vi "Get Status.vi"(8 "error in (no error)":errorcluster, 10 "Header Contents in":T1={"FILENAME"=["FILENAME", "example.fits", "File name at acquisition"], "OBSERVER"=["OBSERVER", "ECHARPE", "PI name"], "PROGRID"=["PROGRID", "UNDEFINED", "Program ID"], "OBJECT"=["OBJECT", "UNDEFINED", "Object name"], "NIGHTDIR"=["NIGHTDIR", "C:\\Users\\Sparc4_2\\Desktop\\Software Echarpe\\Imagens", "Night directory name "], "CHANNEL"=["CHANNEL", "RED", "Instrument channel"], "INSTRUME"=["INSTRUME", "ECHARPE", "Instrument"], "NEXPSEQ"=["NEXPSEQ", "1", "Total number of exposures in sequence"], "SEQINDEX"=["SEQINDEX", "1", "Exposure index in the sequence"], "OBSTYPE"=["OBSTYPE", "BIAS", "Image type: OBJECT, BIAS, FLAT, ARC, DARK"], "READMOD"=["READMOD", "Normal", "Read out mode: fast, normal, slow"], "SHUTTER"=["SHUTTER", "CLOSED", "Shutter Mode (OPEN, CLOSED, or AUTO) "], "OPENSHT"=["OPENSHT", "50", "Time to open the shutter (ms) "], "CLOSESHT"=["CLOSESHT", "50", "Time to close the shutter (ms)"], "GAIN"=["GAIN", "3.38", "Gain (e-/ADU)"], "GAINERR "=["GAINERR", "0.05", " Gain error (e-/ADU)"], "RDNOISE"=["RDNOISE", "6.55", "Read noise (e-)"], "RNOISERR"=["RNOISERR", "0.02", "Read noise error (e-)"], "SKYFIBER"=["SKYFIBER", "OFF", "Sky fiber: ON or OFF"], "CALFIBER"=["CALFIBER", "OFF", "Calibration Fiber: ON or OFF"], "UTDATE"=["UTDATE", "2017-10-01T20", "UT date at start of exposure"], "LOCTIME"=["LOCTIME", "2017-10-01T17", "LT date at start of exposure"], "MJD"=["MJD", "58027.500000", "Modified Julian Date at start of exposure"], "OBSLON"=["OBSLON", "-45.57972", "Observatory East Longitude"], "OBSLAT"=["OBSLAT", "-22.53444", "Observatory Latitude"], "OBSALT"=["OBSALT", "1864.0", "Observatory elevation above sea level (m)"], "EXPTIME"=["EXPTIME", "1", "Exposure time (s)"], "TELRA"=["TELRA", "00:00:00.000", "TCS right ascension: HH:MM:SS.SSS"], "TELDEC"=["TELDEC", "+00:00:00.000", "TCS declination: +-DD:MM:SS.SSS"], "RA"=["RA", "00:00:00.000", "Requested right Ascension: HH:MM:SS.SSS"], "DEC"=["DEC", "+00:00:00.000", "Requested Declination: +- DD:MM:SS.SSS"], "RA_DEG"=["RA_DEG", "128.84946", "Requested Right Ascension (deg)"], "DEC_DEG"=["DEC_DEG", "+19.648717", "Requested Declination (deg)"], "EPOCH"=["EPOCH", "2000.00", "Epoch for Target coordinates"], "HA"=["HA", "+01:13:05.98", "Hour Angle (Sexagesimal)"], "HAD"=["HAD", "1.2183292", "Hour Angle (deg)"], "AIRMASS"=["AIRMASS", "1.085", "Mean airmass for the observation"], "AMSTART"=["AMSTART", "1.060", "Airmass at start of exposure"], "AMEND"=["AMEND", "1.114", "Airmass at end of exposure"], "XOFFSET"=["XOFFSET", "0.000000", "Telescope RA offset in arcsec"], "YOFFSET"=["YOFFSET", "0.000000", "Telescope DEC offset in arcsec"], "PA"=["PA", "14.6415392418", "Current Rotator Position Angle (degree)"], "CAMFOC"=["CAMFOC", "-3.53", "Camera focus position (mm)"], "TELFOC"=["TELFOC", "-3.53", "Telescope focus position (mm)"], "TCSUT"=["TCSUT", "23:17:24.8", "TCS Universal Time"], "MOONDIST"=["MOONDIST", "60.0", "Moon angular distance to object (deg)"], "MOONALT"=["MOONALT", "15.0", "Moon elevation above horizon (deg)"], "MONNPHAS"=["MOONPHAS", "30.0", "Moon phase (deg)"], "ADC"=["ADC", "ON", "Atmospheric Dispersion Corrector: ON or OFF"], "ADCSPPED"=["ADCSPPED", "5.0", "ADC motor speed (rpm)"], "CALMIRR"=["CALMIRR", "OUT", "Calibration mirror position: IN or OUT"], "GUIDING"=["GUIDING", "ON", "Guider status: ON or OFF"], "GUIDTEXP"=["GUIDTEXP", "1.0", "Guider exposure time (s)"], "GUIDFREQ"=["GUIDFREQ", "1.0", "Guiding frequency (Hz)"], "GUIDOBJX"=["GUIDOBJX", "102.5", "Guiding object x position (pixel)"], "GUIDOBJY"=["GUIDOBJY", "300.3", "Guiding object y position (pixel)"], "AVGYCORR"=["AVGYCORR", "2.3", "Average correction in RA (arcsec)"], "AVGXCORR"=["AVGXCORR", "1.3", "Average correction in DEC (arcsec)"], "GFOCUS"=["GFOCUS", "3.0", "Guider focus position (mm)"], "THARLAMP"=["THARLAMP", "OFF", "Thorium-Argon lamp state: ON or OFF"], "HALLAMP"=["HALLAMP", "OFF", "Halogen lamp state: ON or OFF"], "AGITATOR"=["AGITATOR", "ON", "Fiber agitator: ON or OFF"], "THARMIRR"=["THARMIRR", "SPECTROGRAPH", "Th-Ar mirror position: SPECTROGRAPH or TELESCOPE"], "DSTATUS"=["DSTATUS", "OPEN", "Dome Status: OPEN or CLOSED"], "DTEMP"=["DTEMP", "10.0", "Dome temperature (deg C)"], "DHUM"=["DHUM", "82.0", "Dome humidity (per cent)"], "DLAMP"=["DLAMP", "OFF", "Dome lamp: ON or OFF"], "DFLAT"=["DFLAT", "OFF", "Dome flat lamp: ON or OFF"], "TEMPEXT"=["TEMPEXT", "10.0", "External temperature (deg C)"], "PRESSURE"=["PRESSURE", "742.00", "Pressure (mbar)"], "HUMIDITY"=["HUMIDITY", "92.00", "Humidity (per cent)"], "WINDDIR"=["WINDDIR", "15.0", "Wind direction: North-eastward (deg)"], "WSPEED"=["WSPEED", "30.2", "Wind Speed (km/h)"], "TCSST"=["TCSST", "23:12:32.5", "TCS Sideral Time"], "DPOS"=["DPOS", "0.00000", "Dome position (deg)"]}, 11 "Dome in":refnum<class "Dome.lvclass">) -> (0 "error out":errorcluster, 2 "Header Contents out":T1={"FILENAME"=["FILENAME", "example.fits", "File name at acquisition"], "OBSERVER"=["OBSERVER", "ECHARPE", "PI name"], "PROGRID"=["PROGRID", "UNDEFINED", "Program ID"], "OBJECT"=["OBJECT", "UNDEFINED", "Object name"], "NIGHTDIR"=["NIGHTDIR", "C:\\Users\\Sparc4_2\\Desktop\\Software Echarpe\\Imagens", "Night directory name "], "CHANNEL"=["CHANNEL", "RED", "Instrument channel"], "INSTRUME"=["INSTRUME", "ECHARPE", "Instrument"], "NEXPSEQ"=["NEXPSEQ", "1", "Total number of exposures in sequence"], "SEQINDEX"=["SEQINDEX", "1", "Exposure index in the sequence"], "OBSTYPE"=["OBSTYPE", "BIAS", "Image type: OBJECT, BIAS, FLAT, ARC, DARK"], "READMOD"=["READMOD", "Normal", "Read out mode: fast, normal, slow"], "SHUTTER"=["SHUTTER", "CLOSED", "Shutter Mode (OPEN, CLOSED, or AUTO) "], "OPENSHT"=["OPENSHT", "50", "Time to open the shutter (ms) "], "CLOSESHT"=["CLOSESHT", "50", "Time to close the shutter (ms)"], "GAIN"=["GAIN", "3.38", "Gain (e-/ADU)"], "GAINERR "=["GAINERR", "0.05", " Gain error (e-/ADU)"], "RDNOISE"=["RDNOISE", "6.55", "Read noise (e-)"], "RNOISERR"=["RNOISERR", "0.02", "Read noise error (e-)"], "SKYFIBER"=["SKYFIBER", "OFF", "Sky fiber: ON or OFF"], "CALFIBER"=["CALFIBER", "OFF", "Calibration Fiber: ON or OFF"], "UTDATE"=["UTDATE", "2017-10-01T20", "UT date at start of exposure"], "LOCTIME"=["LOCTIME", "2017-10-01T17", "LT date at start of exposure"], "MJD"=["MJD", "58027.500000", "Modified Julian Date at start of exposure"], "OBSLON"=["OBSLON", "-45.57972", "Observatory East Longitude"], "OBSLAT"=["OBSLAT", "-22.53444", "Observatory Latitude"], "OBSALT"=["OBSALT", "1864.0", "Observatory elevation above sea level (m)"], "EXPTIME"=["EXPTIME", "1", "Exposure time (s)"], "TELRA"=["TELRA", "00:00:00.000", "TCS right ascension: HH:MM:SS.SSS"], "TELDEC"=["TELDEC", "+00:00:00.000", "TCS declination: +-DD:MM:SS.SSS"], "RA"=["RA", "00:00:00.000", "Requested right Ascension: HH:MM:SS.SSS"], "DEC"=["DEC", "+00:00:00.000", "Requested Declination: +- DD:MM:SS.SSS"], "RA_DEG"=["RA_DEG", "128.84946", "Requested Right Ascension (deg)"], "DEC_DEG"=["DEC_DEG", "+19.648717", "Requested Declination (deg)"], "EPOCH"=["EPOCH", "2000.00", "Epoch for Target coordinates"], "HA"=["HA", "+01:13:05.98", "Hour Angle (Sexagesimal)"], "HAD"=["HAD", "1.2183292", "Hour Angle (deg)"], "AIRMASS"=["AIRMASS", "1.085", "Mean airmass for the observation"], "AMSTART"=["AMSTART", "1.060", "Airmass at start of exposure"], "AMEND"=["AMEND", "1.114", "Airmass at end of exposure"], "XOFFSET"=["XOFFSET", "0.000000", "Telescope RA offset in arcsec"], "YOFFSET"=["YOFFSET", "0.000000", "Telescope DEC offset in arcsec"], "PA"=["PA", "14.6415392418", "Current Rotator Position Angle (degree)"], "CAMFOC"=["CAMFOC", "-3.53", "Camera focus position (mm)"], "TELFOC"=["TELFOC", "-3.53", "Telescope focus position (mm)"], "TCSUT"=["TCSUT", "23:17:24.8", "TCS Universal Time"], "MOONDIST"=["MOONDIST", "60.0", "Moon angular distance to object (deg)"], "MOONALT"=["MOONALT", "15.0", "Moon elevation above horizon (deg)"], "MONNPHAS"=["MOONPHAS", "30.0", "Moon phase (deg)"], "ADC"=["ADC", "ON", "Atmospheric Dispersion Corrector: ON or OFF"], "ADCSPPED"=["ADCSPPED", "5.0", "ADC motor speed (rpm)"], "CALMIRR"=["CALMIRR", "OUT", "Calibration mirror position: IN or OUT"], "GUIDING"=["GUIDING", "ON", "Guider status: ON or OFF"], "GUIDTEXP"=["GUIDTEXP", "1.0", "Guider exposure time (s)"], "GUIDFREQ"=["GUIDFREQ", "1.0", "Guiding frequency (Hz)"], "GUIDOBJX"=["GUIDOBJX", "102.5", "Guiding object x position (pixel)"], "GUIDOBJY"=["GUIDOBJY", "300.3", "Guiding object y position (pixel)"], "AVGYCORR"=["AVGYCORR", "2.3", "Average correction in RA (arcsec)"], "AVGXCORR"=["AVGXCORR", "1.3", "Average correction in DEC (arcsec)"], "GFOCUS"=["GFOCUS", "3.0", "Guider focus position (mm)"], "THARLAMP"=["THARLAMP", "OFF", "Thorium-Argon lamp state: ON or OFF"], "HALLAMP"=["HALLAMP", "OFF", "Halogen lamp state: ON or OFF"], "AGITATOR"=["AGITATOR", "ON", "Fiber agitator: ON or OFF"], "THARMIRR"=["THARMIRR", "SPECTROGRAPH", "Th-Ar mirror position: SPECTROGRAPH or TELESCOPE"], "DSTATUS"=["DSTATUS", "OPEN", "Dome Status: OPEN or CLOSED"], "DTEMP"=["DTEMP", "10.0", "Dome temperature (deg C)"], "DHUM"=["DHUM", "82.0", "Dome humidity (per cent)"], "DLAMP"=["DLAMP", "OFF", "Dome lamp: ON or OFF"], "DFLAT"=["DFLAT", "OFF", "Dome flat lamp: ON or OFF"], "TEMPEXT"=["TEMPEXT", "10.0", "External temperature (deg C)"], "PRESSURE"=["PRESSURE", "742.00", "Pressure (mbar)"], "HUMIDITY"=["HUMIDITY", "92.00", "Humidity (per cent)"], "WINDDIR"=["WINDDIR", "15.0", "Wind direction: North-eastward (deg)"], "WSPEED"=["WSPEED", "30.2", "Wind Speed (km/h)"], "TCSST"=["TCSST", "23:12:32.5", "TCS Sideral Time"], "DPOS"=["DPOS", "0.00000", "Dome position (deg)"]}, 3 "Dome out":refnum<class "Dome.lvclass">)   [LabVIEW 2018, in "Dome.lvclass"]
uses:
  Dome.lvclass
  Dome.lvclass/Dome.ctl
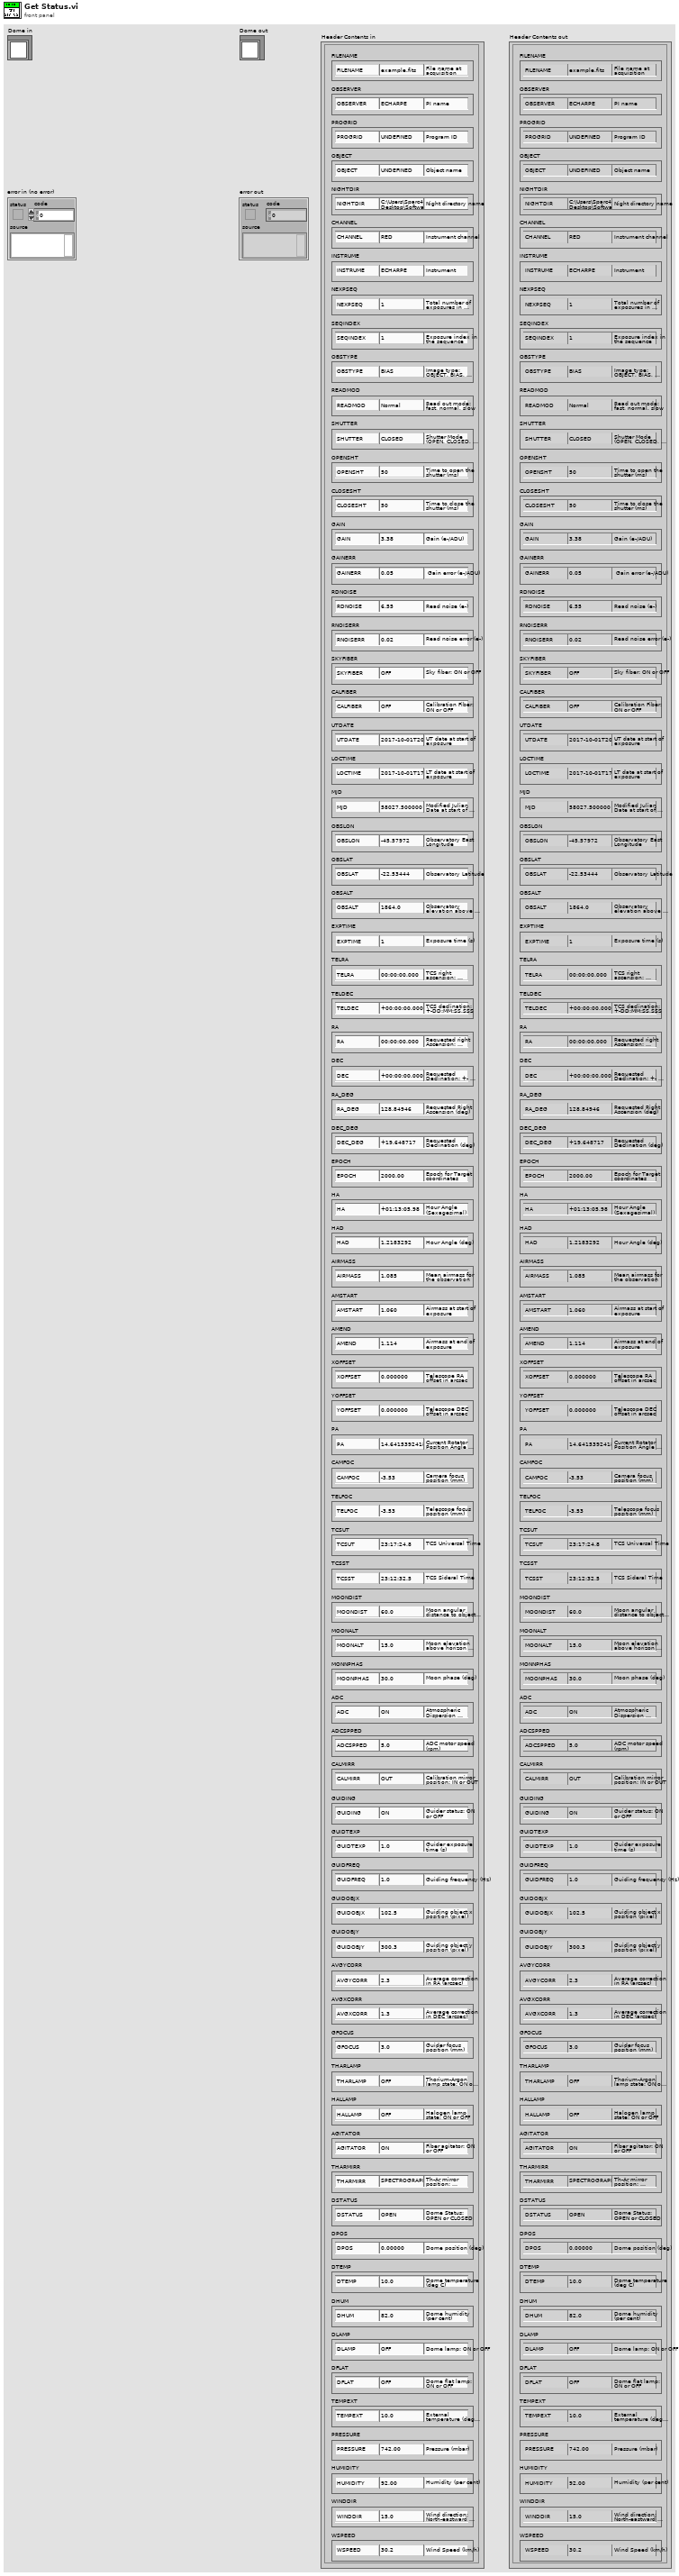
[diagram p1: front panel]
types:
  T1 = cluster{"FILENAME":string[], "OBSERVER":string[], "PROGRID":string[], "OBJECT":string[], "NIGHTDIR":string[], "CHANNEL":string[], "INSTRUME":string[], "NEXPSEQ":string[], "SEQINDEX":string[], "OBSTYPE":string[], "READMOD":string[], "SHUTTER":string[], "OPENSHT":string[], "CLOSESHT":string[], "GAIN":string[], "GAINERR ":string[], "RDNOISE":string[], "RNOISERR":string[], "SKYFIBER":string[], "CALFIBER":string[], "UTDATE":string[], "LOCTIME":string[], "MJD":string[], "OBSLON":string[], "OBSLAT":string[], "OBSALT":string[], "EXPTIME":string[], "TELRA":string[], "TELDEC":string[], "RA":string[], "DEC":string[], "RA_DEG":string[], "DEC_DEG":string[], "EPOCH":string[], "HA":string[], "HAD":string[], "AIRMASS":string[], "AMSTART":string[], "AMEND":string[], "XOFFSET":string[], "YOFFSET":string[], "PA":string[], "CAMFOC":string[], "TELFOC":string[], "TCSUT":string[], "MOONDIST":string[], "MOONALT":string[], "MONNPHAS":string[], "ADC":string[], "ADCSPPED":string[], "CALMIRR":string[], "GUIDING":string[], "GUIDTEXP":string[], "GUIDFREQ":string[], "GUIDOBJX":string[], "GUIDOBJY":string[], "AVGYCORR":string[], "AVGXCORR":string[], "GFOCUS":string[], "THARLAMP":string[], "HALLAMP":string[], "AGITATOR":string[], "THARMIRR":string[], "DSTATUS":string[], "DTEMP":string[], "DHUM":string[], "DLAMP":string[], "DFLAT":string[], "TEMPEXT":string[], "PRESSURE":string[], "HUMIDITY":string[], "WINDDIR":string[], "WSPEED":string[], "TCSST":string[], "DPOS":string[]}
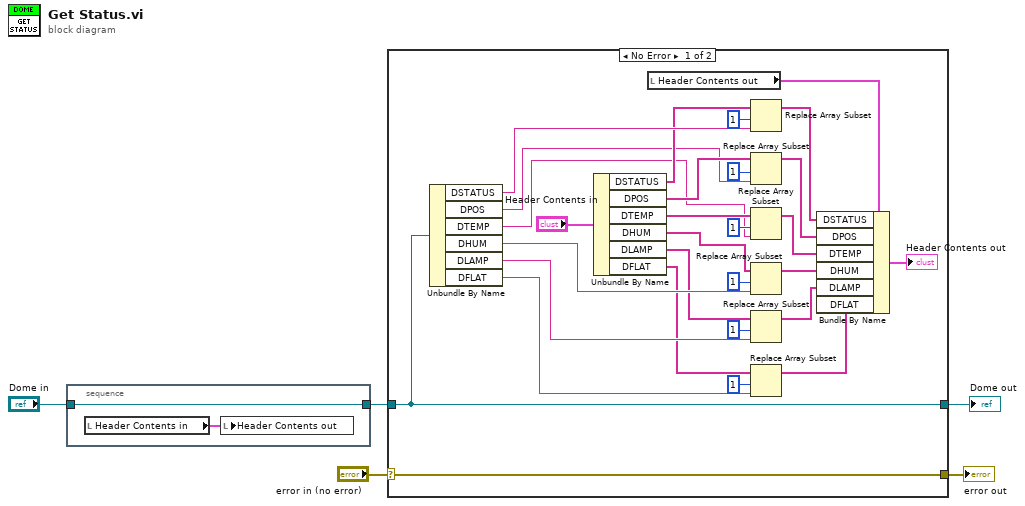
[diagram p0: block diagram]
diagram:
  n1 = stacked-sequence {
    tunnel: "Dome in" -> [w6]
    tunnel: [w6] -> w5
    frame #0 {
      n2 = local read "Header Contents in"() -> (w7:T1)
      n3 = local write "Header Contents out"(w7) -> ()
    }
  }
  n4 = case shown="No Error" "error in (no error)" {
    selector: "error in (no error)" -> [w36 w38]
    tunnel: [w36 w38] -> w3
    tunnel: [w26 w37] -> w1
    tunnel: w5 -> [w26 w37]
    frame No Error {
      n5 = Unbundle By Name(w26) -> ("DSTATUS"=w25:string, "DPOS"=w9:string, "DTEMP"=w8:string, "DHUM"=w22:string, "DLAMP"=w23:string, "DFLAT"=w24:string)
      n6 = Unbundle By Name("Header Contents in") -> ("DSTATUS"=w21:string[], "DPOS"=w20:string[], "DTEMP"=w19:string[], "DHUM"=w11:string[], "DLAMP"=w10:string[], "DFLAT"=w18:string[])
      n7 = local read "Header Contents out"() -> (w30:T1)
      n8 = Replace Array Subset(array=w21, new element=w25, index=1) -> (w17:string[])
      n9 = Replace Array Subset(array=w20, new element=w9, index=1) -> (w16:string[])
      n10 = Replace Array Subset(array=w19, new element=w8, index=1) -> (w15:string[])
      n11 = Replace Array Subset(array=w11, new element=w22, index=1) -> (w14:string[])
      n12 = Replace Array Subset(array=w10, new element=w23, index=1) -> (w13:string[])
      n13 = Replace Array Subset(array=w18, new element=w24, index=1) -> (w12:string[])
      n14 = Bundle By Name(cluster=w30, "DSTATUS"=w17, "DPOS"=w16, "DTEMP"=w15, "DHUM"=w14, "DLAMP"=w13, "DFLAT"=w12) -> (→"Header Contents out":T1)
    }
    frame Error {
    }
  }
  "error out" <- w3
  "Dome out" <- w1
